vi "Model - Get CNTRLR States.vi"(8 "error in (no error)":errorcluster, 11 "View Model":T2) -> (0 "error out":errorcluster, 1 "Next State":T1, 2 "Current State":T1, 3 "View Model":T2)   [LabVIEW 2017]
doc: "Get actual CNTRLR States Values from DVR."
uses:
  Controls/View Model.ctl
  Controls/Shared Model.ctl
  Error Handler/Controls/Error Model.ctl
  Error Handler/Controls/Error Message.ctl
  Error Handler/Controls/Error Level.ctl
  Configuration/Controls/Database Model.ctl
  Configuration/Controls/Database Message.ctl
  Configuration/Controls/Database Command.ctl
  Configuration/Controls/Database Overhead.ctl
  Configuration/Controls/Database Status.ctl
  Configuration/Controls/Database Record.ctl
  Configuration/Controls/Database - Rule Record.ctl
  Controller/Controls/CNTRLR - Wash Step.ctl
  Controller/Controls/CNTRLR - Position.ctl
  Controller/Controls/CNTRLR - Model.ctl
  Controller/Controls/CNTRLR - Message.ctl
  Controller/Controls/CNTRLR - Command.ctl
  Controller/Controls/CNTRLR - Overhead.ctl
  Controller/Controls/CNTRLR - State.ctl
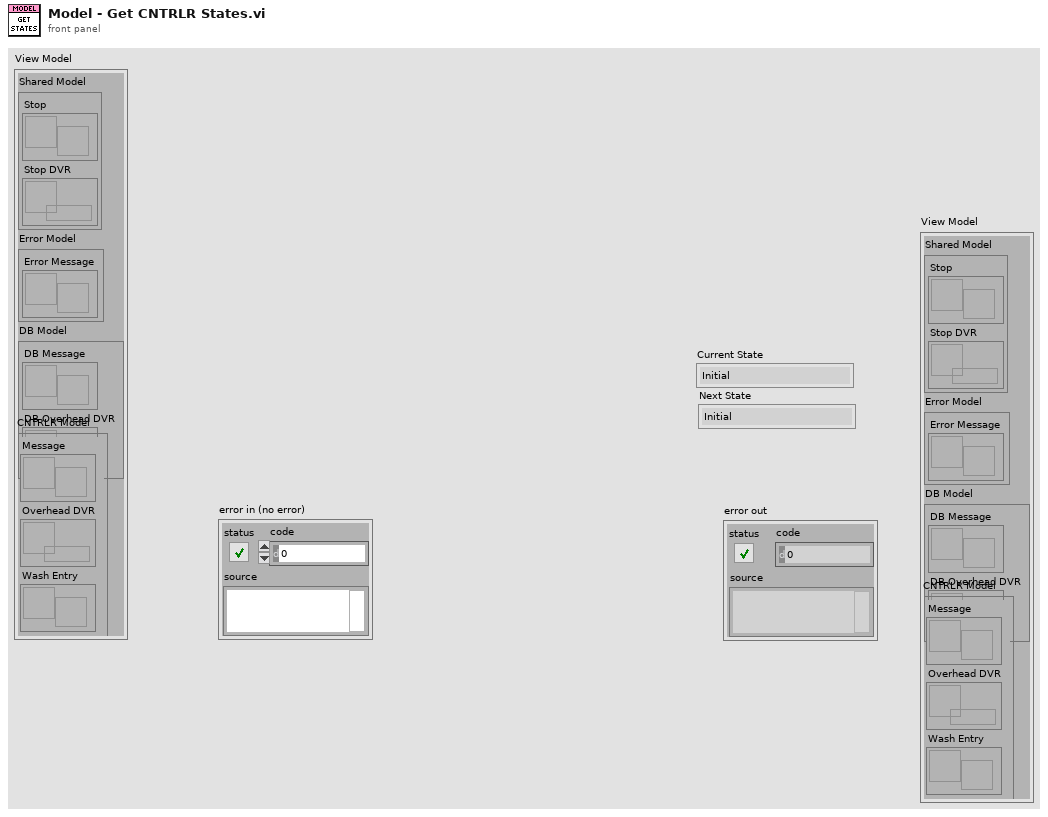
[diagram p1: front panel]
types:
  T1 = typedef "CNTRLR - State.ctl" = enum16{"Initial", "Wait for Start", "Start State", "Wait for Vehicle Position", "Wash Step Execution", "Wash Step/Cycle Complete", "Wash Exit", "Wash Abort/Terminate"}
  T2 = typedef "View Model.ctl" = cluster{"Shared Model":T3, "Error Model":T4, "DB Model":T5, "CNTRLR Model":T6}
  T3 = typedef "Shared Model.ctl" = cluster{"Stop":refnum<user-event>, "Stop DVR":refnum<data-value>}
  T4 = typedef "Error Model.ctl" = cluster{"Error Message":refnum<user-event>}
  T5 = typedef "Database Model.ctl" = cluster{"DB Message":refnum<user-event>, "DB Overhead DVR":refnum<data-value>}
  T6 = typedef "CNTRLR - Model.ctl" = cluster{"Message":refnum<user-event>, "Overhead DVR":refnum<data-value>, "Wash Entry":refnum<user-event>, "Out of Position":refnum<user-event>}
  T7 = typedef "CNTRLR - Overhead.ctl" = cluster{"Vehicle Position":T8, "Current State":T1, "Next State":T1, "Wash Cycle":T9[], "Current Wash Step":T10, "Time Remaining":dbl}
  T8 = typedef "CNTRLR - Position.ctl" = enum16{"Entry", "Station 1", "Station 2", "Station 3", "Exit"}
  T9 = typedef "Database Record.ctl" = cluster{"Wash Step":string, "Station":string, "Step Duration":u32}
  T10 = typedef "CNTRLR - Wash Step.ctl" = enum16{"Under Body Wash", "Bug Remover", "Pre-Soak", "High Pressure Wash", "Low Pressure Wax", "Spot Free Rinse", "Tire Shine Foam", "Air Dry", "None"}
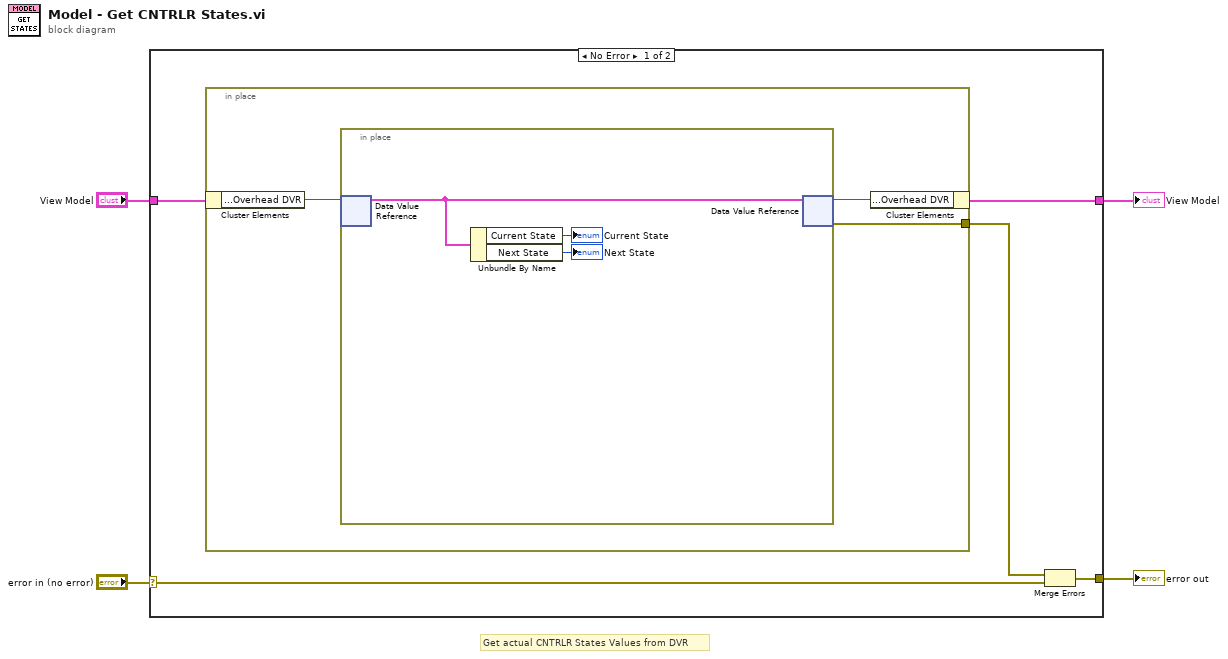
[diagram p0: block diagram]
diagram:
  # "Get actual CNTRLR States Values from DVR"
  n1 = case shown="No Error" "error in (no error)" {
    selector: "error in (no error)" -> [w7 w17]
    tunnel: [w5 w17] -> w3
    tunnel: "View Model" -> [w9 w16]
    tunnel: [w8 w16] -> w1
    frame No Error {
      n2 = in-place {
        in-place-border: [w10] -> w6
        n3 = in-place-cluster #1(w9) -> ("CNTRLR Model.Overhead DVR"=w12:refnum<data-value>)
        n4 = in-place {
          n5 = in-place-dvr #2(w12) -> (w15:T7)  [unwired: 1 out]
          n6 = Unbundle By Name(w15) -> ("Current State"=→"Current State":T1, "Next State"=→"Next State":T1)
          n7 = in-place-dvr #2(w15) -> (w11:refnum<data-value>, w10:errorcluster)
        }
        n8 = in-place-cluster #1("CNTRLR Model.Overhead DVR"=w11) -> (w8:T2)
      }
      n9 = Merge Errors(w6, w7) -> (w5:errorcluster)
    }
    frame Error {
      # "If any Error occurred do nothing"
    }
  }
  "error out" <- w3
  "View Model" <- w1
